vi "AlliGator Update Phasor Graph Information at Cursor.vi"(6 "Valid?":bool, 8 "Error In":errorcluster, 9 "Phasor SDV":T1={"g"=nan, "s"=nan}, 10 "Phasor":T1, 11 "Current Phasor Information Indicators":T2) -> (0 "Error Out":errorcluster, 3 "Phase Lifetime":dbl[unit])   [LabVIEW 2021, in "AlliGator Phasor Graph.lvlib"]
doc: "Computes phasor-related quantities and displays them in the Phasor Graph panel."
uses:
  AlliGator Phasor Graph.lvlib
  AlliGator Phasor Graph Ctrl Refnums.ctl
  Phasor/Phasor Calibration Type.ctl
  Phasor/Phasor (g, s).ctl
  AlliGator Settings List.ctl
  Phasor/Phasor Ratio Type.ctl
  Phasor/Phasor Standard Deviation Options.ctl
  Phasor/Phasor.lvlib
  AlliGator Settings.lvlib
  AlliGator Phasor Ratio.lvlib
  AlliGator GUI.lvlib
panel:
  # "see the AlliGator License on the block diagram (Ctrl+E or Window:Show Block Diagram)"
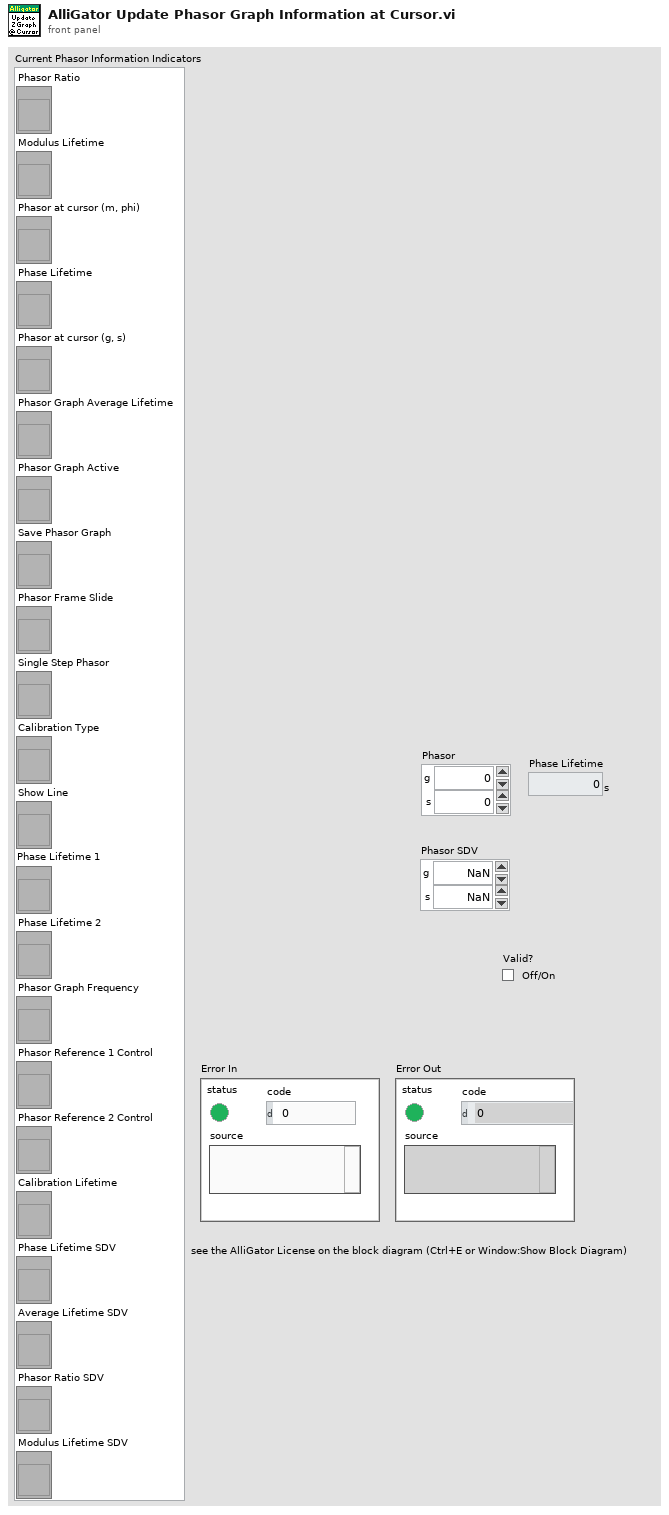
[diagram p1: front panel]
types:
  T1 = typedef "Phasor.lvlib/Phasor (g, s).ctl" = cluster{"g":dbl, "s":dbl}
  T2 = typedef "AlliGator GUI.lvlib/AlliGator Phasor Graph Ctrl Refnums.ctl" = cluster{"Phasor Ratio":refnum<vi>, "Modulus Lifetime":refnum<vi>, "Phasor at cursor (m, phi)":refnum<vi>, "Phase Lifetime":refnum<vi>, "Phasor at cursor (g, s)":refnum<vi>, "Phasor Graph Average Lifetime":refnum<vi>, "Phasor Graph Active":refnum<vi>, "Save Phasor Graph":refnum<vi>, "Phasor Frame Slide":refnum<vi>, "Single Step Phasor":refnum<vi>, "Calibration Type":refnum<vi>, "Show Line":refnum<vi>, "Phase Lifetime 1":refnum<vi>, "Phase Lifetime 2":refnum<vi>, "Phasor Graph Frequency":refnum<vi>, "Phasor Reference 1 Control":refnum<vi>, "Phasor Reference 2 Control":refnum<vi>, "Calibration Lifetime":refnum<vi>, "Phase Lifetime SDV":refnum<vi>, "Average Lifetime SDV":refnum<vi>, "Phasor Ratio SDV":refnum<vi>, "Modulus Lifetime SDV":refnum<vi>}
  T3 = typedef "Phasor.lvlib/Phasor Standard Deviation Options.ctl" = cluster{"Compute Estimated SDV":bool, "# Replicas":u32, "Use Estimated Average Phasor":bool}
  T4 = typedef "AlliGator Settings.lvlib/AlliGator Settings List.ctl" = enum16{"GUI:Visible Settings Tab", "GUI:Last Run Version", "Source Image:Use Image Histogram for Contrast", "Source Image:Low Count Pixels Rejection Options", "Source Image:High Count Pixels Rejection Options", "Source Image:Use Image Brightness", "Source Image:Blend Overlay with Image Background", "Source Image:Use Fixed ROI Diameter", "Source Image:ROI Diameter", "Source Image:ROI Center Color", "Source Image:Peak Threshold", "Source Image:Intensity Threshold", "Source Image:Image Binning Options", "Source Image:Image Smoothing Options", "Source Image:Image Histogram Active", "Source Image:Invert Binary Mask", "Source Image:Hot Pixel Removal", "Source Image:Overlay Analyzed ROI Center", "Source Image:Auto-Adjust Contrast", "Source Image:Histogram Lower Percentile", "Source Image:Histogram Upper Percentile", "Source Image:Save Source Image", "Source Image:Scale Bar Options", "Source Image:Image Resolution (Pixel Size)", "Source Image:Flatfield Correction", "Source Image:Show Dead Left Columns Correction", "Source Image:Dead Left Columns Correction", "Source Image:Image Pre-Processing Operations Order", "Data Information:Gate Width", "Data Information:Nanotime Gate Separation", "Data Information:Macrotime Gate Separation", "Data Information:Gate Step", "Data Information:# Gates", "Data Information:Gate Image Exposure", "Data Information:Gate Image Integration", "Data Information:Gates to Skip", "Data Information:Gates to Keep", "Data Information:Define Gates to", "Data Information:Channel Name", "Data Information:Available Channel Names", "Data Information:Channel Arithmetic", "Data Information:Background File Subtraction", "Data Information:Background File", "Data Information:Background Scaling Factor", "Data Information:Background Pile-up Correction", "Data Information:Background Pixel Well Capacity", "Data Information:Laser Period", "Data Information:SYNC Period", "Data Information:Pile-up Correction", "Data Information:Pixel Well Capacity", "Data Information:Dataset Scaling Factor", "Fluorescence Decay_Decay Pre-Processing:Reverse Gates", "Fluorescence Decay_Decay Pre-Processing:Verbose Decay Pre-Processing", "Fluorescence Decay_Decay Pre-Processing:Use Decay Pre-Processing", "Fluorescence Decay_Decay Pre-Processing:Background Subtraction", "Fluorescence Decay_Decay Pre-Processing:Background Definition Range", "Fluorescence Decay_Decay Pre-Processing:Baseline Subtraction Method", "Fluorescence Decay_Decay Pre-Processing:Decay Pre-Processing Operations Order", "Fluorescence Decay_Decay Pre-Processing:Smoothing Parameter", "Fluorescence Decay_Decay Pre-Processing:Shift Decay", "Fluorescence Decay_Decay Pre-Processing:Decay Shift Parameters", "Fluorescence Decay_Decay Pre-Processing:Fold Decay", "Fluorescence Decay_Decay Pre-Processing:# Folds", "Fluorescence Decay_Decay Pre-Processing:1-Normalize Decay", "Fluorescence Decay_Decay Pre-Processing:[0-1]-Normalize Decay", "Fluorescence Decay_Decay Pre-Processing:Smoothen Decay", "Fluorescence Decay_Decay Pre-Processing:Extrapolate Decay", "Fluorescence Decay_Decay Pre-Processing:Use Periodicity", "Fluorescence Decay_Decay Pre-Processing:Use Cursors", "Fluorescence Decay_Decay Pre-Processing:Tail Fraction", "Fluorescence Decay_Decay Pre-Processing:Head Fraction", "Fluorescence Decay_Decay Pre-Processing:Additional Points", "Fluorescence Decay_Decay Pre-Processing:Straighten Decay", "Fluorescence Decay_Decay Pre-Processing:Constant Background", "Fluorescence Decay_Decay Pre-Processing:Pixel-Normalize Decay", "Fluorescence Decay_Advanced Analysis:Extract IRF instead of Decay", "Fluorescence Decay_Advanced Analysis:IRF Extraction Options", "Fluorescence Decay_Advanced Analysis:IRF Optimization Options", "Fluorescence Decay_Advanced Analysis:Square Pulse Options", "Fluorescence Decay_Advanced Analysis:IRF Order", "Fluorescence Decay_Advanced Analysis:IRF Time Constants", "Fluorescence Decay_Advanced Analysis:Wavelet Analysis Options", "Fluorescence Decay_Advanced Analysis:Average Lifetime Options", "Fluorescence Decay_Fit Options:Fit Options", "Fluorescence Decay_Fit Options:Use Legacy Fitting Approach", "Fluorescence Decay_Fit Options:Use Data Information Laser Period", "Fluorescence Decay_Fit Parameters:Displayed Fit Parameters", "Fluorescence Decay_Fit Parameters:Fit Parameter Constraints", "Fluorescence Decay_Fit Parameters:Export Tabulated Results", "Fluorescence Decay_Fit Parameters:MLE Baseline Offset Type", "Fluorescence Decay_Fit Parameters:MLE Baseline Offset", "Fluorescence Decay_Fit Parameters:Guess Parameter Names", "Fluorescence Decay_Fit Parameters:Guess Parameter Values", "Fluorescence Decay_Fit Parameters:Guess Parameters Options", "Fluorescence Decay_Styles:Show Last Decay Only", "Fluorescence Decay_Styles:Decay Graph Color Array", "Fluorescence Decay:Decay Graph Active", "Fluorescence Decay Statistics:Min Peak Value", "Fluorescence Decay Statistics:Reject Low Decay Peak Pixels", "Fluorescence Decay Statistics:Reject High Decay Peak Pixels", "Fluorescence Decay Statistics:Max Peak Value", "Time Traces:Use File Timestamp", "Time Traces:Time Step", "Time Traces:Use Intensity Correction File", "Time Traces:Intensity Correction File", "Phasor Plot:Phasor Plot Smoothing Options", "Phasor Plot:Phasor Plot Size", "Phasor Plot:Phasor Plot Graphics Options", "Phasor Plot:Cumulative Phasor Plot", "Phasor Plot:Use Phasor Brightness", "Phasor Plot:Blend Overlay with Phasor Background", "Phasor Plot:Save Phasor Plot", "Phasor Plot:Show References", "Phasor Plot:Phasor Ratio Decay Range", "Phasor Plot:Exponential Fading", "Phasor Plot:Phasor Ratio Reference Colors", "Phasor Plot:Reference Radius", "Phasor Plot:Show Color Map Vertices", "Phasor Plot:Phasor Plot Active", "Phasor Plot:Phasor Ratio Color Map Type", "Phasor Plot:Phasor Ratio Color Map", "Phasor Plot:Phasor Ratio Display Range", "Phasor Plot:Selected Image ROI(s)", "Phasor Plot:All Image ROIs", "Phasor Plot:Selected Phasor Plot ROI(s)", "Phasor Plot:All Phasor Plot ROIs", "Phasor Plot:Phasor Ratio Color-Coded Quantity", "Phasor Plot:Store Phasor Harmonics", "Phasor Plot:Draw Reference Segment", "Phasor Plot:User-Defined Quantity", "Phasor Graph:Phasor Frequency", "Phasor Graph:Phasor Ratio Type", "Phasor Graph:Pixel-level Phasor Computation", "Phasor Graph:Save Phasor Graph", "Phasor Graph:Phasor Graph Active", "Phasor Graph:Phasor SDV Options", "Phasor Calibration:Use Backup Calibration if needed", "Phasor Graph:Define Shortest Lifetime as", "Phasor Calibration:Backup Calibration Type", "Phasor Calibration:Calibration Type", "Phasor Calibration:Calibration Lifetime", "Phasor Calibration:Calibration Map Algorithm", "Single-Exponential Phasor Locus (SEPL):Gate Parameters", "Single-Exponential Phasor Locus (SEPL):User-defined Gate", "Single-Exponential Phasor Locus (SEPL):User-defined IRF", "Single-Exponential Phasor Locus (SEPL):Phasor Parameters", "Single-Exponential Phasor Locus (SEPL):Decay & IRF Parameters", "Single-Exponential Phasor Locus (SEPL):Display Parameters", "Lifetime Analysis:Decay Analysis Parameters", "Lifetime Analysis:Lifetime Map Active", "Plugins:Python Settings", "Miscellaneous:Verbose Mode", "Miscellaneous:Beep after Script", "Miscellaneous:Saved Image File Format", "Miscellaneous:Exported Gate Image Settings", "Miscellaneous:Include Loading in Timing", "Miscellaneous:Verbose Settings Mode", "Miscellaneous:Histogram Options", "Miscellaneous:Beep on Error", "Miscellaneous:# Logical Processors Used", "Miscellaneous:ROI Description Max Characters", "Miscellaneous:Verbose Error Mode", "Miscellaneous:Transparent Mask Color"}
  T5 = typedef "Phasor.lvlib/Phasor Ratio Type.ctl" = enum32{"Intensity-weighted", "Amplitude-weighted"}
  T6 = typedef "Phasor.lvlib/Phasor (m, phi).ctl" = cluster{"m":dbl, "phi":dbl}
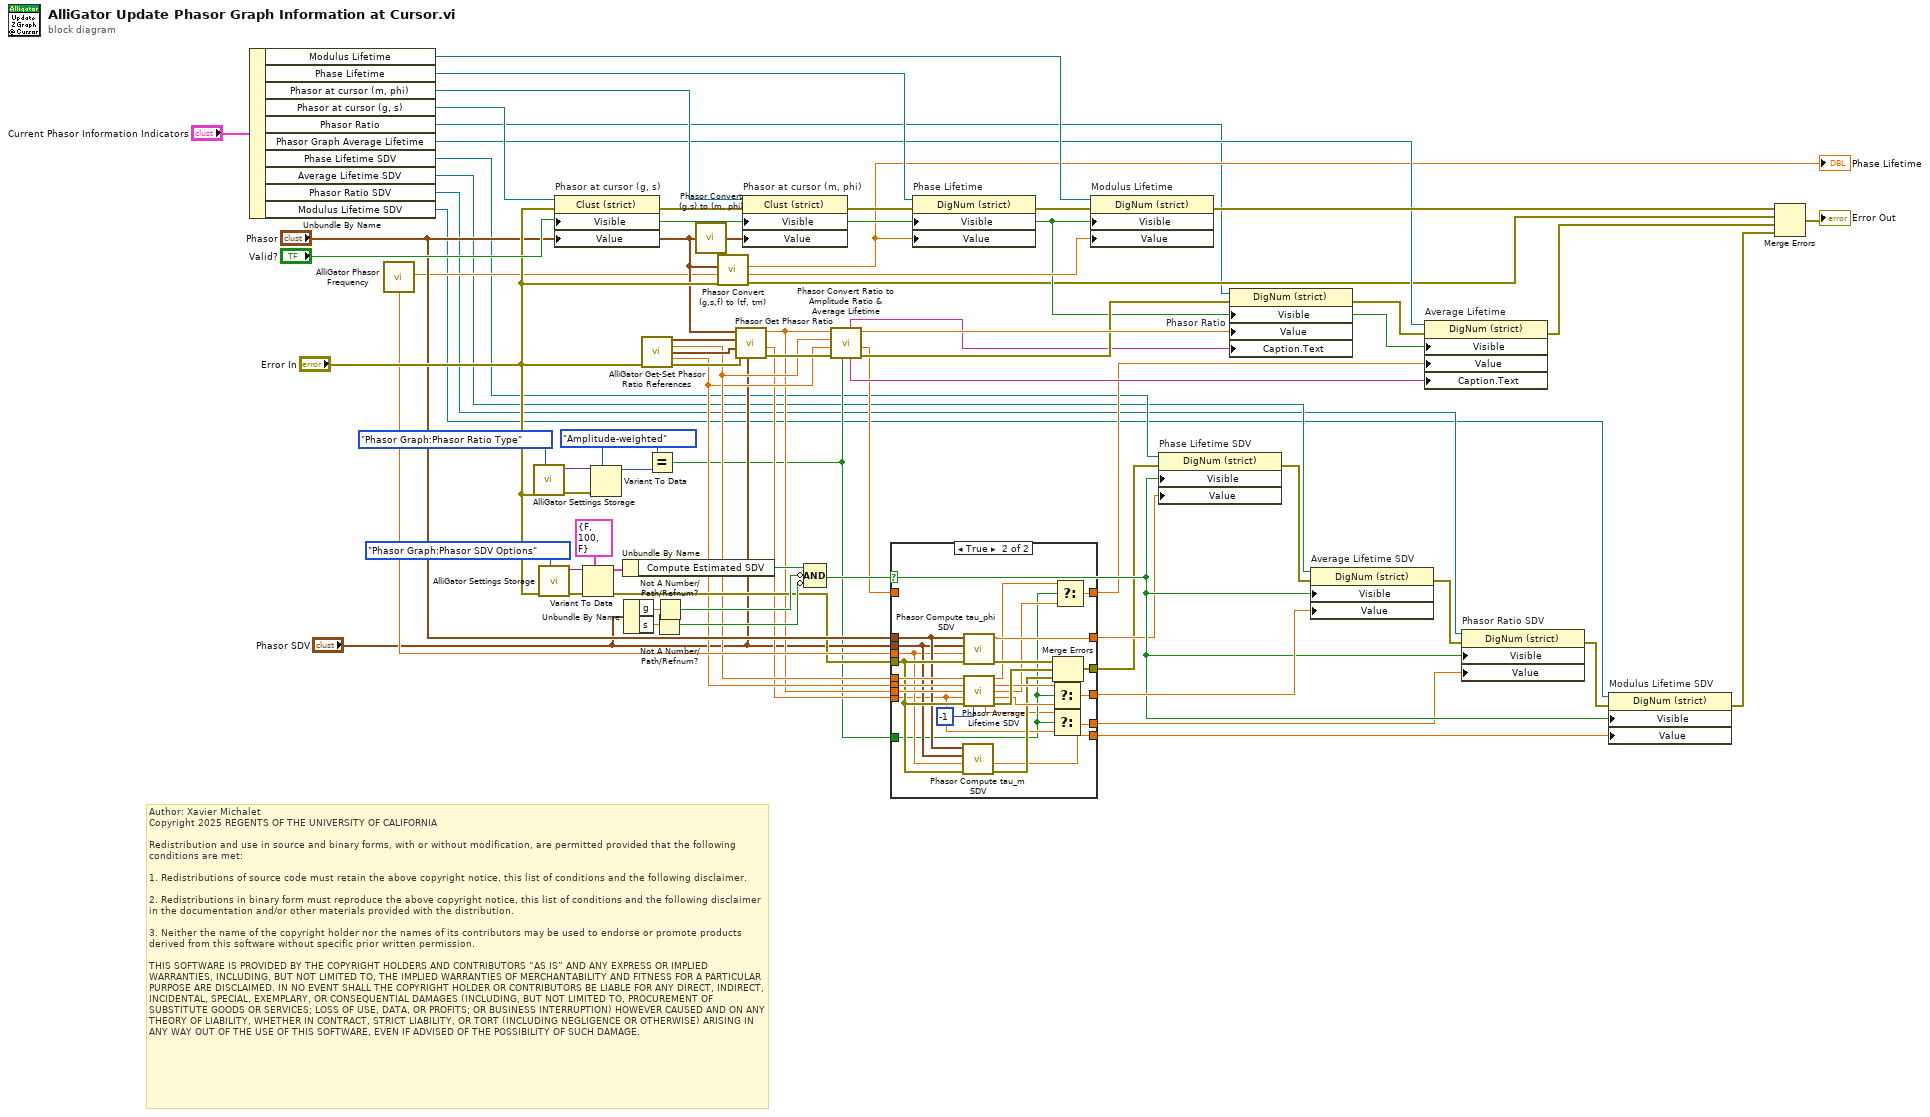
[diagram p0: block diagram]
diagram:
  w43 = Phasor_Ratio_Type."Amplitude-weighted" ("Phasor Ratio Type")
  # "Author: Xavier Michalet\nCopyright 2025 REGENTS OF THE UNIVERSITY OF CALIFORNIA\n\nRedistribution and use in source and binary forms, with or without modification, are permitted provided that the following conditions are met:\n\n1. Redistributions of source code must retain the above copyright notice, this list of conditions and the following disclaimer.\n\n2. Redistributions in binary form must reproduce the above copyright notice, this list of conditions and the following disclaimer in the documentation and/or other materials provided with the distribution.\n\n3. Neither the name of the copyright holder nor the names of its contributors may be used to endorse or promote products derived from this software without specific prior written permission.\n\nTHIS SOFTWARE IS PROVIDED BY THE COPYRIGHT HOLDERS AND CONTRIBUTORS “AS IS” AND ANY EXPRESS OR IMPLIED WARRANTIES, INCLUDING, BUT NOT LIMITED TO, THE IMPLIED WARRANTIES OF MERCHANTABILITY AND FITNESS FOR A PARTICULAR PURPOSE ARE DISCLAIMED. IN NO EVENT SHALL THE COPYRIGHT HOLDER OR CONTRIBUTORS BE LIABLE FOR ANY DIRECT, INDIRECT, INCIDENTAL, SPECIAL, EXEMPLARY, OR CONSEQUENTIAL DAMAGES (INCLUDING, BUT NOT LIMITED TO, PROCUREMENT OF SUBSTITUTE GOODS OR SERVICES; LOSS OF USE, DATA, OR PROFITS; OR BUSINESS INTERRUPTION) HOWEVER CAUSED AND ON ANY THEORY OF LIABILITY, WHETHER IN CONTRACT, STRICT LIABILITY, OR TORT (INCLUDING NEGLIGENCE OR OTHERWISE) ARISING IN ANY WAY OUT OF THE USE OF THIS SOFTWARE, EVEN IF ADVISED OF THE POSSIBILITY OF SUCH DAMAGE."
  n1 = Unbundle By Name("Current Phasor Information Indicators") -> ("Modulus Lifetime"=w54:refnum<vi>, "Phase Lifetime"=w57:refnum<vi>, "Phasor at cursor (m, phi)"=w58:refnum<vi>, "Phasor at cursor (g, s)"=w59:refnum<vi>, "Phasor Ratio"=w30:refnum<vi>, "Phasor Graph Average Lifetime"=w49:refnum<vi>, "Phase Lifetime SDV"=w4:refnum<vi>, "Average Lifetime SDV"=w3:refnum<vi>, "Phasor Ratio SDV"=w2:refnum<vi>, "Modulus Lifetime SDV"=w1:refnum<vi>)
  n2 = call "AlliGator Phasor Frequency.vi"() -> ("Phasor Frequency"=w18:dbl[unit])
  n3 = call "AlliGator Settings Storage.vi"("AlliGator Settings List"=AlliGator_Settings_List."Phasor Graph:Phasor Ratio Type", "Error In"="Error In") -> ("Error Out"=w41:errorcluster, "Variant Data out"=w42:variant)  [unwired: 8 in]
  n4 = call "AlliGator Settings Storage.vi"("AlliGator Settings List"=AlliGator_Settings_List."Phasor Graph:Phasor SDV Options", "Error In"="Error In") -> ("Error Out"=w38:errorcluster, "Variant Data out"=w39:variant)  [unwired: 8 in]
  n5 = property on="Phasor at cursor (g, s)" class="Clust (strict)"(reference=w59, error in="Error In", "Visible"="Valid?", "Value"="Phasor") -> (error out=w63:errorcluster)  [unwired: 1 out]
  n6 = Variant To Data(error in=w38, type=T3 {"Compute Estimated SDV"=FALSE, "# Replicas"=100, "Use Estimated Average Phasor"=FALSE} ("Phasor SDV Options"), Variant=w39) -> (data=w36:T3, error out=w17:errorcluster)
  n7 = Variant To Data(error in=w41, type=w43, Variant=w42) -> (data=w44:T5)  [unwired: 1 out]
  n8 = Unbundle By Name(w36) -> ("Compute Estimated SDV"=w35:bool)
  n9 = Unbundle By Name("Phasor SDV") -> ("g"=w24:dbl, "s"=w23:dbl)
  n10 = call "AlliGator Get-Set Phasor Ratio References.vi"("error in (no error)"="Error In") -> ("Reference Phasor 1"=w65:T1, "Reference Lifetime 1"=w15:dbl[unit], "Reference Phasor 2"=w66:T1, "Reference Lifetime 2"=w14:dbl[unit], "error out"=w67:errorcluster)  [unwired: 7 in, 3 out]
  n11 = Equal?(x=w43, y=w44) -> (x = y?=w7:bool)
  n12 = Not A Number/Path/Refnum?(number/path/refnum=w23) -> (NaN/Path/Refnum?=w20:bool)
  n13 = Not A Number/Path/Refnum?(number/path/refnum=w24) -> (NaN/Path/Refnum?=w21:bool)
  n14 = call "Phasor Convert (g,s) to (m, phi).vi"("Phasor (g, s)"="Phasor") -> ("Phasor (m, phi)"=w62:T6)  [unwired: 8 in]
  n15 = call "Phasor Convert (g,s,f) to (tf, tm).vi"("Error In"="Error In", "Phasor Harmonic Frequency"=w18, "Phasor (g, s)"="Phasor") -> ("Error Out"=w31:errorcluster, "Modulus Lifetime"=w61:dbl[unit], "Phase Lifetime"=w32:dbl[unit])  [unwired: 6 in]
  "Phase Lifetime" <- w32
  n16 = call "Phasor Get Phasor Ratio.vi"("Phasor SDV"="Phasor SDV", "Error In"=w67, "Reference Phasor 2"=w66, "Reference Phasor 1"=w65, "Phasor"="Phasor") -> ("Error Out"=w64:errorcluster, "Phasor Ratio SDV"=w12:dbl, "Phasor Ratio (f1)"=w9:dbl)  [unwired: 4 in]
  n17 = property on="Phasor at cursor (m, phi)" class="Clust (strict)"(reference=w58, error in=w63, "Visible"="Valid?", "Value"=w62) -> (error out=w56:errorcluster)  [unwired: 1 out]
  n18 = Compound Arithmetic op=AND(w35, invert w21, invert w20) -> (w22:bool)
  n19 = call "Phasor Convert Ratio to Amplitude Ratio & Average Lifetime.vi"("Compute Amplitude Ratio"=w7, "error in (no error)"=w64, "Reference Lifetime 2"=w14, "Reference Lifetime 1"=w15, "Phasor Ratio (f1)"=w9) -> ("error out"=w53:errorcluster, "Average Lifetime"=w6:dbl[unit], "Phasor/Amplitude Ratio"=w68:dbl, "Average Lifetime Caption"=w46:string, "Phasor Ratio Plot Name Suffix"=w50:string)  [unwired: 2 in]
  n20 = case shown="True" w22 {
    tunnel: [_ w85] -> w34
    tunnel: [_ w94] -> w16
    tunnel: "Phasor" -> [_ w81]
    tunnel: "Phasor SDV" -> [_ w80]
    tunnel: w18 -> [_ w79]
    tunnel: w17 -> [w70 w84]
    tunnel: w15 -> [_ w93]
    tunnel: w14 -> [_ w92]
    tunnel: [w70 w89] -> w13
    tunnel: w12 -> [_ w74]
    tunnel: [_ w75] -> w11
    tunnel: [_ w82] -> w10
    tunnel: w9 -> [_ w88]
    tunnel: w7 -> [_ w73]
    tunnel: w6 -> [w69 _]
    tunnel: [w69 w76] -> w5
    frame False {
    }
    frame True {
      n21 = call "Phasor Compute tau_m SDV.vi"("Error In"=w84, "Phasor Frequency"=w79, "Phasor SDV (g, s)"=w80, "Phasor (g, s)"=w81) -> ("Error Out"=w83:errorcluster, "tau_m SDV"=w82:dbl[unit])  [unwired: 5 in, 1 out]
      n22 = call "Phasor Compute tau_phi SDV.vi"("Error In"=w84, "Phasor Frequency"=w79, "Phasor SDV (g, s)"=w80, "Phasor (g, s)"=w81) -> ("Error Out"=w91:errorcluster, "tau_phi SDV"=w94:dbl[unit])  [unwired: 6 in]
      n23 = call "Phasor Average Lifetime SDV.vi"("tau 1"=w93, "tau 2"=w92, "r"=w88, "SDV r"=w74, "Error In"=w84, "seed"=-1) -> ("<tau>_a"=w78:dbl[unit], "SDV <tau>_a"=w87:dbl[unit], "<tau>_i"=w77:dbl[unit], "SDV <tau>_i"=w86:dbl[unit], "SDV a"=w72:dbl, "Error Out"=w90:errorcluster)  [unwired: 4 in]
      n24 = Select(t=w87, s=w73, f=w86) -> (s? t:f=w85:dbl[unit])
      n25 = Select(t=w72, s=w73, f=w74) -> (s? t:f=w75:dbl)
      n26 = Merge Errors(w91, w90, w83) -> (w89:errorcluster)
      n27 = Select(t=w78, s=w73, f=w77) -> (s? t:f=w76:dbl[unit])
    }
  }
  n28 = property on="Phase Lifetime" class="DigNum (strict)"(reference=w57, error in=w56, "Visible"="Valid?", "Value"=w32) -> (error out=w55:errorcluster)  [unwired: 1 out]
  n29 = property on="Modulus Lifetime" class="DigNum (strict)"(reference=w54, error in=w55, "Visible"="Valid?", "Value"=w61) -> (error out=w52:errorcluster)  [unwired: 1 out]
  n30 = property on="Phase Lifetime SDV" class="DigNum (strict)"(reference=w4, error in=w13, "Visible"=w22, "Value"=w16) -> (error out=w29:errorcluster)  [unwired: 1 out]
  n31 = property on="Phasor Ratio" class="DigNum (strict)"(reference=w30, error in=w53, "Visible"="Valid?", "Value"=w68, "Caption.Text"=w50) -> (error out=w48:errorcluster)  [unwired: 1 out]
  n32 = property on="Average Lifetime SDV" class="DigNum (strict)"(reference=w3, error in=w29, "Visible"=w22, "Value"=w34) -> (error out=w28:errorcluster)  [unwired: 1 out]
  n33 = property on="Average Lifetime" class="DigNum (strict)"(reference=w49, error in=w48, "Visible"="Valid?", "Value"=w5, "Caption.Text"=w46) -> (error out=w47:errorcluster)  [unwired: 1 out]
  n34 = property on="Phasor Ratio SDV" class="DigNum (strict)"(reference=w2, error in=w28, "Visible"=w22, "Value"=w11) -> (error out=w27:errorcluster)  [unwired: 1 out]
  n35 = property on="Modulus Lifetime SDV" class="DigNum (strict)"(reference=w1, error in=w27, "Visible"=w22, "Value"=w10) -> (error out=w25:errorcluster)  [unwired: 1 out]
  n36 = Merge Errors(w52, w31, w47, w25) -> (→"Error Out":errorcluster)
